vi "custom message2.vi"(10 "Boolean":bool, 11 "Numeric":i32) -> ()   [LabVIEW 2019]
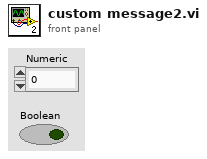
[diagram p1: front panel]
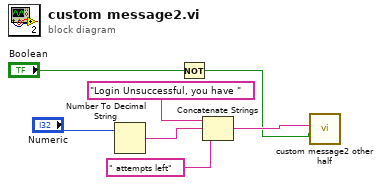
[diagram p0: block diagram]
diagram:
  n1 = Number To Decimal String(number="Numeric") -> (decimal integer string=w6:string)  [unwired: 1 in]
  n2 = Not(x="Boolean") -> (.not. x?=w1:bool)
  n3 = Concatenate Strings("Login Unsuccessful, you have " ("string"), w6, " attempts left" ("string")) -> (w2:string)
  n4 = call "custom message2 other half.vi"("Enable"=w1, "Message"=w2) -> ()  [unwired: 8 in, 2 out]
